vi "XNET Database Create (LIN Schedule Entry).vi"(0 "LIN schedule in":refnum<k21>, 7 "LIN schedule entry name":string, 11 "error in (no error)":errorcluster) -> (4 "LIN schedule out":refnum<k21>, 8 "LIN schedule entry out":refnum<k21>, 15 "error out":errorcluster)   [LabVIEW 2018]
doc: "Creates a new LIN schedule entry."
uses:
  nixlvapi.dll
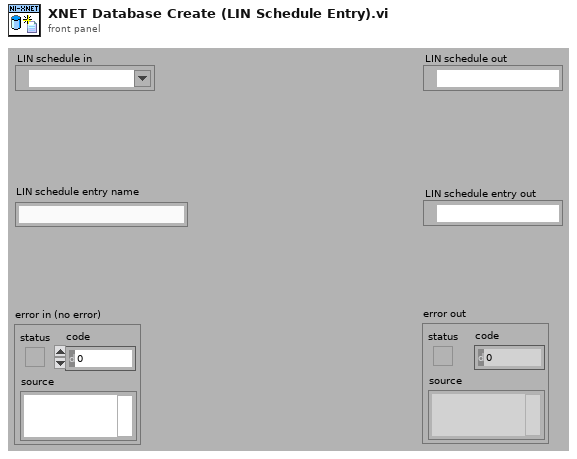
[diagram p1: front panel]
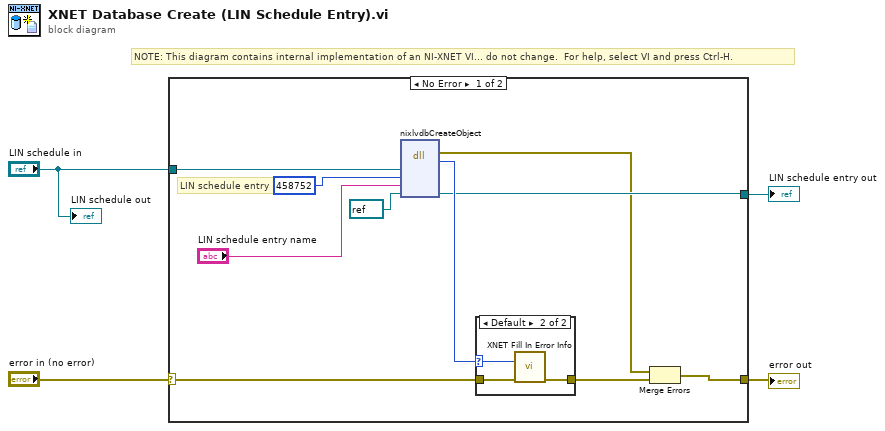
[diagram p0: block diagram]
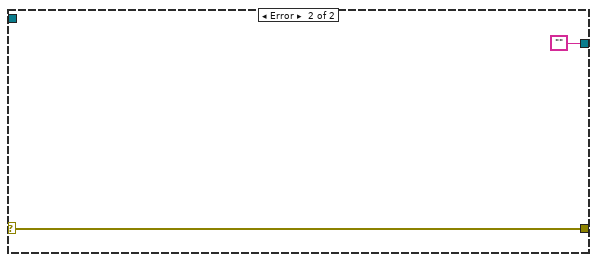
[diagram p3: hidden frame]
diagram:
  # "NOTE: This diagram contains internal implementation of an NI-XNET VI... do not change.  For help, select VI and press Ctrl-H."
  n1 = case shown="No Error" "error in (no error)" {
    selector: "error in (no error)" -> [w14 w20]
    tunnel: [w6 w20] -> w4
    tunnel: [w7 ""] -> w1
    tunnel: "LIN schedule in" -> [w9 _]
    frame No Error {
      # "LIN schedule entry"
      n2 = dll-call lib="nixlvapi.*" fn="nixlvdbCreateObject" ("nilvxaiu.dll:lvxenDatabaseCreateObject")("parentObjRef"=w9, "objectClass"=u32 458752 ("class"), "objectName"="LIN schedule entry name", refnum<k21> refnum ("LIN schedule entry out")) -> (error out=w5:errorcluster, "return type"=w13:i32, w7:refnum<k21>)  [unwired: 5 in, 2 out]
      n3 = case shown="Default" w13 {
        selector: w13 -> [_ w16]
        tunnel: w14 -> [w15 w17]
        tunnel: [w15 w18] -> w12
        frame 0 {
        }
        frame Default {
          n4 = call "XNET Fill In Error Info.vi"("status code"=w16, "error in"=w17) -> ("error out"=w18:errorcluster)  [unwired: 13 out]
        }
      }
      n5 = Merge Errors(w5, w12) -> (w6:errorcluster)
    }
    frame Error {
    }
  }
  "error out" <- w4
  "LIN schedule entry out" <- w1
  "LIN schedule out" <- "LIN schedule in"
